vi "LJM_eWriteAddresses Example.vi"() -> (0 "error out":errorcluster)   [LabVIEW 2020]
panel:
  out "Error String":string
  out "ConnectionType Out":i32
  out "DeviceType Out":i32
  in  "Identifier":string="LJM_idANY"
  in  "ConnectionType":string="LJM_ctANY"
  in  "DeviceType":string="LJM_dtANY"
  in  "Values":dbl[](array[numeric])=[2.5, 12345.0] format="%.2f"
  in  "Types":i32[](array[numeric])=[3, 0]
  in  "Addresses":i32[](array[numeric])=[1000, 55110]
  out "ErrorAddress":i32
  # "Common Registers:\nAddress, Name, Type, Read/Write\n0, AIN0, 3, RO\n2, AIN1, 3, RO\n1000, DAC0, 3, RW\n1002, DAC1, 3, RW\n2000, FIO0, 0, RW\n2001, FIO1, 0, RW\n55110, TEST_UINT16, 0, RW\n60000, PRODUCT_ID, 3, RO\n60004, FIRMWARE_VERSION, 3, RO\n60028, SERIAL_NUMBER, 1, RO\n\nTypes: 0=UINT16, 1=UINT32, 2=INT32, 3=FLOAT32"
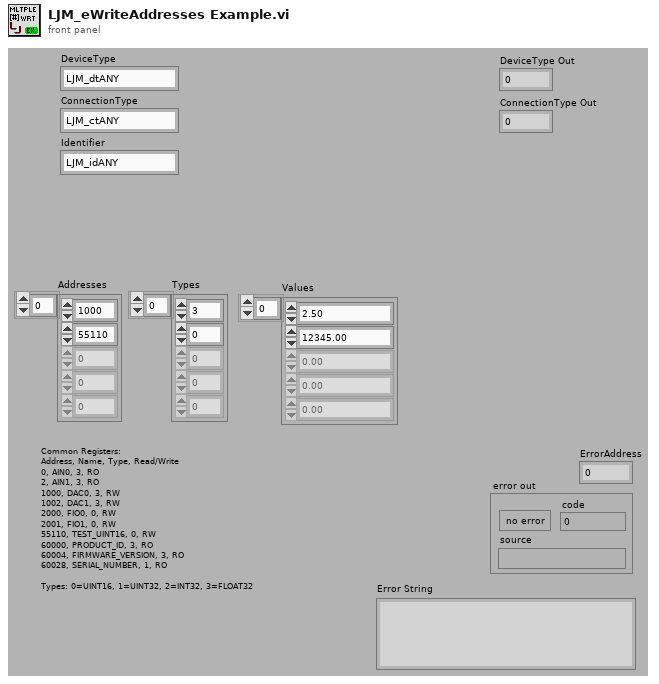
[diagram p1: front panel]
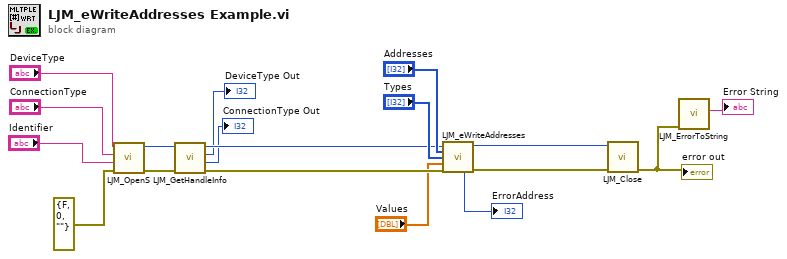
[diagram p0: block diagram]
diagram:
  n1 = call "LJM_OpenS.vi"("error in"=errorcluster {"status"=FALSE, "code"=0, "source"=""} ("error in (no error)"), "Identifier"="Identifier", "ConnectionType"="ConnectionType", "DeviceType"="DeviceType") -> ("error out"=w14:errorcluster, "Handle"=w12:i32)  [unwired: 6 in]
  n2 = call "LJM_GetHandleInfo.vi"("error in"=w14, "Handle In"=w12) -> ("error out"=w13:errorcluster, "ConnectionType"=→"ConnectionType Out":i32, "DeviceType"=→"DeviceType Out":i32, "Handle Out"=w11:i32)  [unwired: 2 in, 4 out]
  n3 = call "LJM_eWriteAddresses.vi"("Handle In"=w11, "aAddresses"="Addresses", "aTypes"="Types", "aValues"="Values", "error in"=w13) -> ("Handle Out"=w10:i32, "ErrorAddress"=→"ErrorAddress":i32, "error out"=w17:errorcluster)  [unwired: 8 in]
  n4 = call "LJM_Close.vi"("error in"=w17, "Handle"=w10) -> ("error out"=w4:errorcluster)  [unwired: 9 in]
  "error out" <- w4
  n5 = call "LJM_ErrorToString.vi"("error in"=w4) -> ("String"=→"Error String":string)  [unwired: 10 in]
